vi "Draw Assert Data.vi"(8 "error in (no error)":errorcluster, 9 "Sort Configuration":T1, 10 "Assert Data":string[][](array[string]), 11 "UserInterface in":refnum<class "UserInterface.lvclass">) -> (0 "error out":errorcluster)   [LabVIEW 2016, in "UserInterface.lvlib" / "UserInterface.lvclass"]
uses:
  UserInterface.lvclass
  Sort Configuration.ctl
  UserInterface.lvclass/UserInterface.ctl
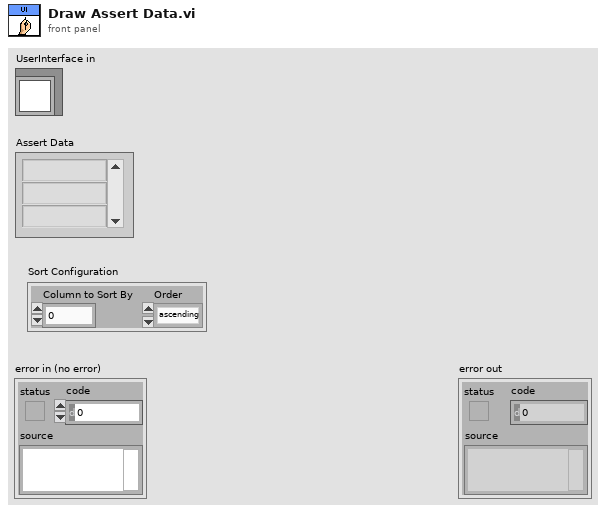
[diagram p1: front panel]
types:
  T1 = typedef "UserInterface.lvlib/UserInterface.lvclass/Sort Configuration.ctl" = cluster{"Column to Sort By":u32, "Order":enum16{"ascending", "descending"}}
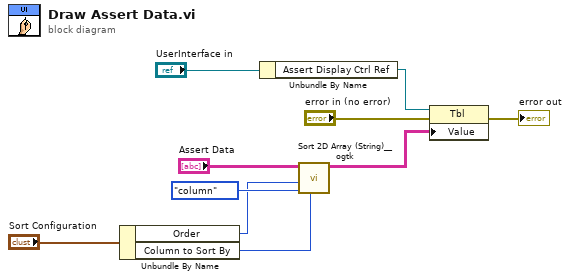
[diagram p0: block diagram]
diagram:
  n1 = Unbundle By Name("Sort Configuration") -> ("Order"=w5:enum16{"ascending", "descending"}, "Column to Sort By"=w6:u32)
  n2 = Unbundle By Name("UserInterface in") -> ("Assert Display Ctrl Ref"=w9:refnum<vi>)
  n3 = call "Sort 2D Array (String)__ogtk.vi"("Column/Row to Sort By"=w6, "Sort By in"=enum16{"row", "column"}."column", "Order"=w5, "Array in"="Assert Data") -> ("Sorted Array out"=w3:string[][])  [unwired: 4 in, 3 out]
  n4 = property class="Tbl"(reference=w9, error in="error in (no error)", "Value"=w3) -> (error out=→"error out":errorcluster)  [unwired: 1 out]
